vi "Add Triggers for Acyclic Frames.vi"(8 "error in":errorcluster, 10 "acyclic frame names":string[](array[string]), 11 "bus controller in":T1 format="%.0x") -> (0 "error out":errorcluster, 3 "bus controller out":T1 format="%.0x")   [LabVIEW 2020, in "Ballard MIL-STD-1553 Scripting.lvlib"]
uses:
  Ballard MIL-STD-1553 Scripting.lvlib
  <vilib>/NI VeriStand/Custom Device API/Custom Device Item Ref.ctl
  Constants.vi
  <vilib>/NI VeriStand/Custom Device API/Custom Device API.lvlib
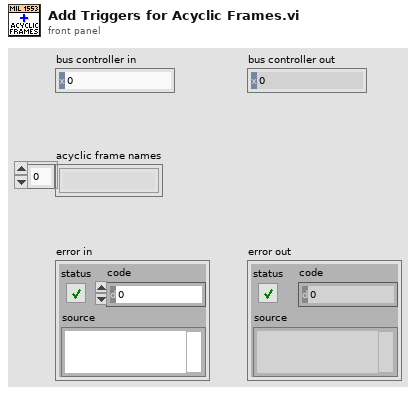
[diagram p1: front panel]
types:
  T1 = typedef "Custom Device API.lvlib/Custom Device Item Ref.ctl" = u64
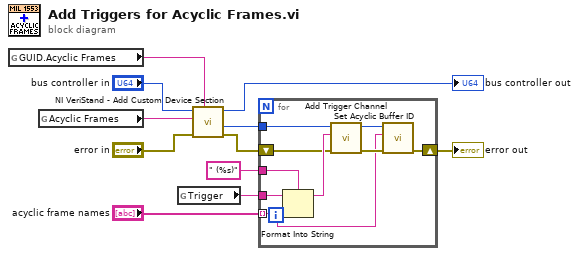
[diagram p0: block diagram]
diagram:
  n1 = global read "Constants.vi" "GUID.Acyclic Frames"() -> (w5:string)
  n2 = global read "Constants.vi" "Acyclic Frames"() -> (w4:string)
  n3 = global read "Constants.vi" "Trigger"() -> (w11:string)
  n4 = call <vilib>:"NI VeriStand - Add Custom Device Section.vi"("GUID (Default Section)"=w5, "error in (no error)"="error in", "Section Name"=w4, "Parent Ref in"="bus controller in") -> ("error out"=w2:errorcluster, "Section Ptr"=w1:T1, "Parent Ref out"=→"bus controller out":T1)  [unwired: 4 in, 1 out]
  n5 = for {
    tunnel: w11 -> [w20]
    tunnel: " (%s)" ("format string") -> [w19]
    shift-right: [w14] -> w9
    shift-left: w2 -> [w17]
    tunnel: "acyclic frame names" -> [w12] mode=indexing
    tunnel: w1 -> [w16]
    n6 = Format Into String(format string=w19, initial string=w20, w12) -> (resulting string=w18:string)  [unwired: 1 in, 1 out]
    n7 = call "Add Trigger Channel.vi"("error in"=w17, "name"=w18, "acyclic frames section"=w16) -> ("error out"=w15:errorcluster, "acyclic frame trigger"=w13:T1)  [unwired: 7 in]
    n8 = call "Set Acyclic Buffer ID.vi"("error in"=w15, "acyclic buffer ID"=w12, "acyclic frame trigger in"=w13) -> ("error out"=w14:errorcluster)  [unwired: 7 in, 1 out]
  }
  "error out" <- w9
